vi "addFile.vi"(8 "error in (no error)":errorcluster, 10 "LV_VGS.lvlib:VGS_VolumeDescriptor+File.lvclass":refnum<class "VGS_VolumeDescriptor+File.lvclass">, 11 "VGS_VolumeDescriptor in":refnum<class "VGS_VolumeDescriptor.lvclass">) -> (0 "error out":errorcluster, 3 "VGS_VolumeDescriptor out":refnum<class "VGS_VolumeDescriptor.lvclass">)   [LabVIEW 2022 SP3, in "LV_VGS.lvlib" / "VGS_VolumeDescriptor.lvclass"]
uses:
  VGS_VolumeDescriptor.lvclass
  VolumeDescriptor+File/VGS_VolumeDescriptor+File.lvclass
  VGS_VolumeDescriptor.lvclass/VGS_VolumeDescriptor.ctl
  C:/Users/Andrey/Desktop/hajo/LV_VGS/vgs_project.dll
  vgs_project.dll
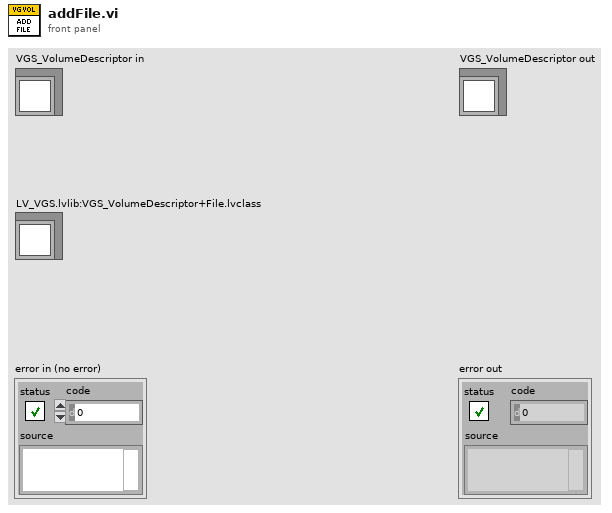
[diagram p1: front panel]
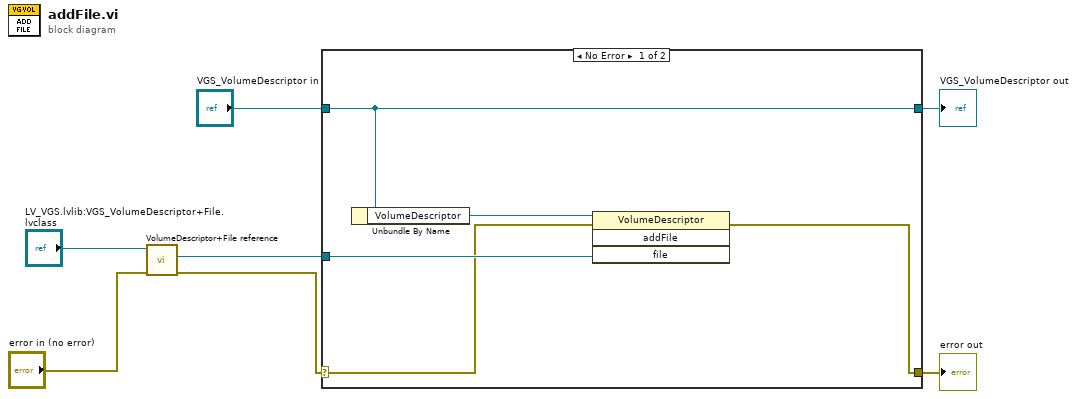
[diagram p0: block diagram]
diagram:
  n1 = call "VolumeDescriptor+File reference.vi"("error in (no error)"="error in (no error)", "VGS_VolumeDescriptor+File in"="LV_VGS.lvlib:VGS_VolumeDescriptor+File.lvclass") -> ("error out"=w1:errorcluster, "VolumeDescriptor+File"=w3:refnum<k24>)  [unwired: 7 in, 1 out]
  n2 = case shown="No Error" w1 {
    selector: w1 -> [w9 w14]
    tunnel: [w8 w14] -> w7
    tunnel: [w12 w13] -> w5
    tunnel: "VGS_VolumeDescriptor in" -> [w12 w13]
    tunnel: w3 -> [w10 _]
    frame No Error {
      n3 = Unbundle By Name(w12) -> ("VolumeDescriptor"=w11:refnum<k24>)
      n4 = invoke class="VolumeDescriptor" method="addFile"(reference=w11, error in=w9, "file"=w10) -> (error out=w8:errorcluster)  [unwired: 1 in, 3 out]
    }
    frame Error {
    }
  }
  "error out" <- w7
  "VGS_VolumeDescriptor out" <- w5
